vi "SystemID.vi"(6 "file path (dialog if empty)":path, 8 "error in":errorcluster, 10 "Value":dbl format="%#_13g", 11 "Time":u32) -> (0 "error out":errorcluster)   [LabVIEW 2012]
uses:
  <vilib>/Utility/file.llb/Write To Spreadsheet File (string).vi
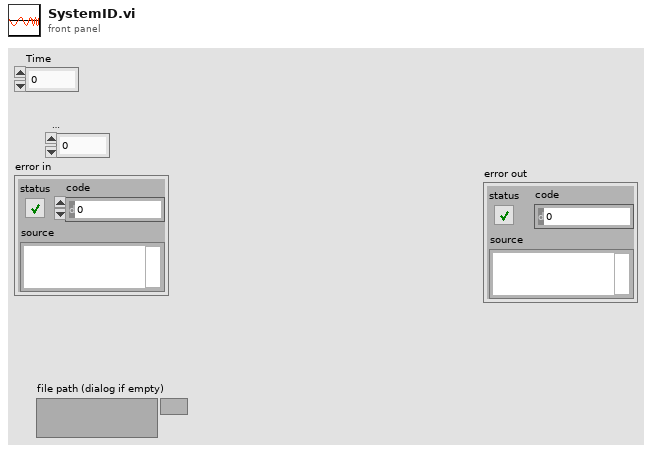
[diagram p1: front panel]
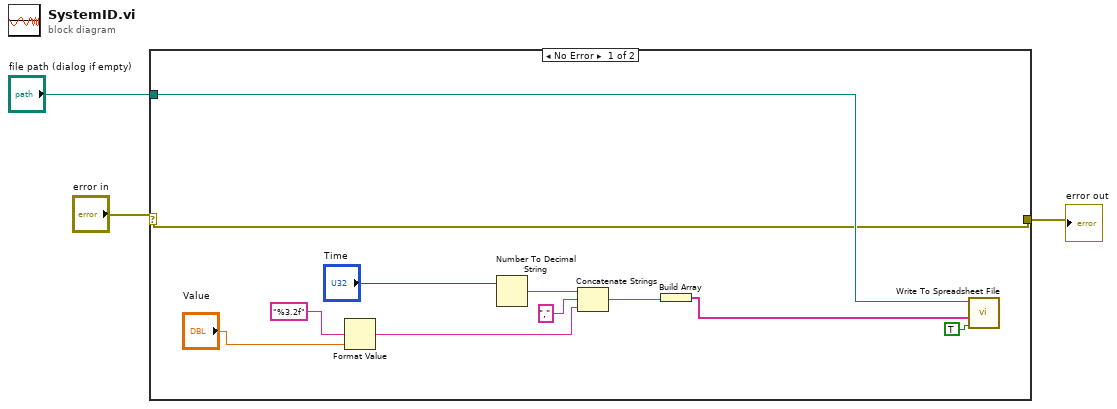
[diagram p0: block diagram]
diagram:
  n1 = case shown="No Error" "error in" {
    selector: "error in" -> [w4 w15]
    tunnel: [w4 w15] -> w2
    tunnel: "file path (dialog if empty)" -> [w7 _]
    frame No Error {
      n2 = Format Value(format string="%3.2f", value (0)="Value") -> (output string=w9:string)  [unwired: 1 in]
      n3 = Number To Decimal String(number="Time") -> (decimal integer string=w8:string)  [unwired: 1 in]
      n4 = Concatenate Strings(w8, "," ("string"), w9) -> (w11:string)
      n5 = Build Array(w11) -> (w10:string[])
      n6 = call-poly <vilib>:"Write To Spreadsheet File.vi"("append to file? (new file:F)"=TRUE, "1D data"=w10, "file path (dialog if empty)"=w7) -> ()  [unwired: 5 in, 1 out]
    }
    frame Error {
    }
  }
  "error out" <- w2
